vi "WriteCommand.vi"(8 "Error In":errorcluster, 10 "Command":string, 11 "Sierra M100 In":refnum<visa-resource-name>) -> (0 "Error Out":errorcluster, 1 "CRC":u16 format="%.0x", 2 "Formatted Command":string, 3 "Sierra M100 Out":refnum<visa-resource-name>)   [LabVIEW 2012, in "Sierra-M100.lvlib"]
doc: "This VI writes the ASCII command string to the serial port. The serial receive buffer is flushed prior to sending the bytes."
uses:
  Sierra-M100.lvlib
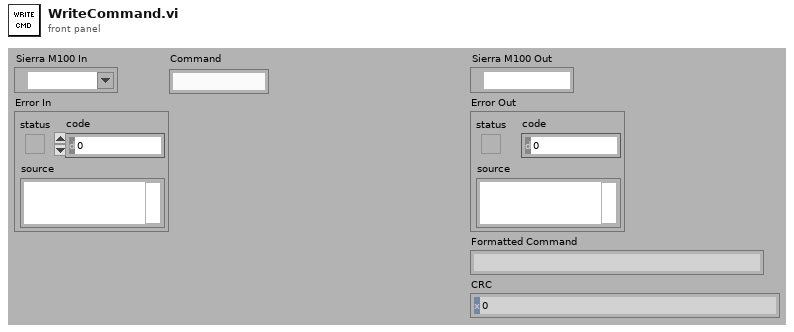
[diagram p1: front panel]
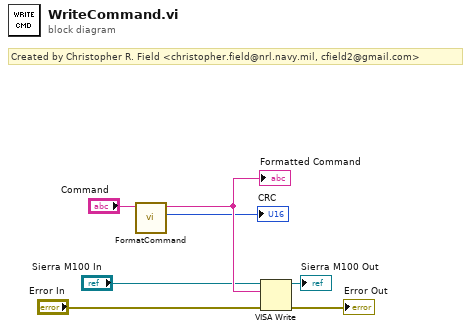
[diagram p0: block diagram]
diagram:
  # "Created by Christopher R. Field <christopher.field@nrl.navy.mil, cfield2@gmail.com>"
  n1 = call "FormatCommand.vi"("Command"="Command") -> ("CRC"=→"CRC":u16, "Formatted Command"=w7:string)  [unwired: 9 in]
  "Formatted Command" <- w7
  n2 = VISA Write(VISA resource name="Sierra M100 In", write buffer=w7, error in (no error)="Error In") -> (VISA resource name out=→"Sierra M100 Out":refnum<visa-resource-name>, error out=→"Error Out":errorcluster)  [unwired: 1 out]
